vi "Facade 1.vi"(0 "Data In":T8, 2 "Display State In":T2={"Item_Refnums_Array"=[], "Root Command"={"Operation"=enum."Add Item", "Data"=variant}}, 3 "Container State":T7) -> (6 "Data Out":T8, 7 "Display State Out":T2={"Item_Refnums_Array"=[], "Root Command"={"Operation"=enum."Add Item", "Data"=variant}}, 8 "Action":T1)   [LabVIEW 2011, in "Root_XControl.xctl"]
uses:
  Root_XControl.xctl
  Data 1.ctl
  <vilib>/_xctls/Container State.ctl
  State 1.ctl
  Controls/References/Item_Refnums.ctl
  Controls/References/Item_Command_Refnum.ctl
  Controls/Item_Command_Enum.ctl
  Controls/Root_Command.ctl
  Controls/Root_Command_Enum.ctl
  <vilib>/_xctls/Action.ctl
  <vilib>/_xctls/XControlSupport.lvlib
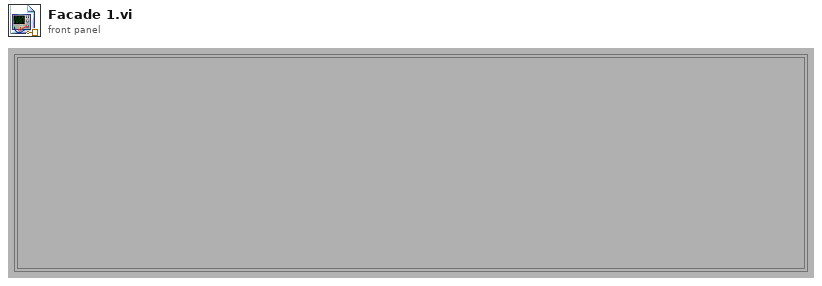
[diagram p1: front panel]
types:
  T1 = typedef "XControlSupport.lvlib/Action.ctl" = cluster{"Data Changed?":bool, "State Changed?":bool, "Action Name":string}
  T2 = typedef "Root_XControl.xctl/State 1.ctl" = cluster{"Item_Refnums_Array":T3[], "Root Command":T5}
  T3 = typedef "Item_Refnums.ctl" = cluster{"VI Refnum":refnum<vi>, "Item_Command_Refnum":T4, "Slide Refnum":refnum<vi>}
  T4 = typedef "Item_Command_Refnum.ctl" = refnum<vi>
  T5 = typedef "Root_Command.ctl" = cluster{"Operation":T6, "Data":variant}
  T6 = typedef "Root_Command_Enum.ctl" = enum16{"Idle", "Add Item", "Delete Item", "Delete All"}
  T7 = typedef "XControlSupport.lvlib/Container State.ctl" = cluster{"Indicator?":bool, "Run Mode?":bool, " Refnum":refnum<vi>}
  T8 = typedef "Root_XControl.xctl/Data 1.ctl" = dbl[]
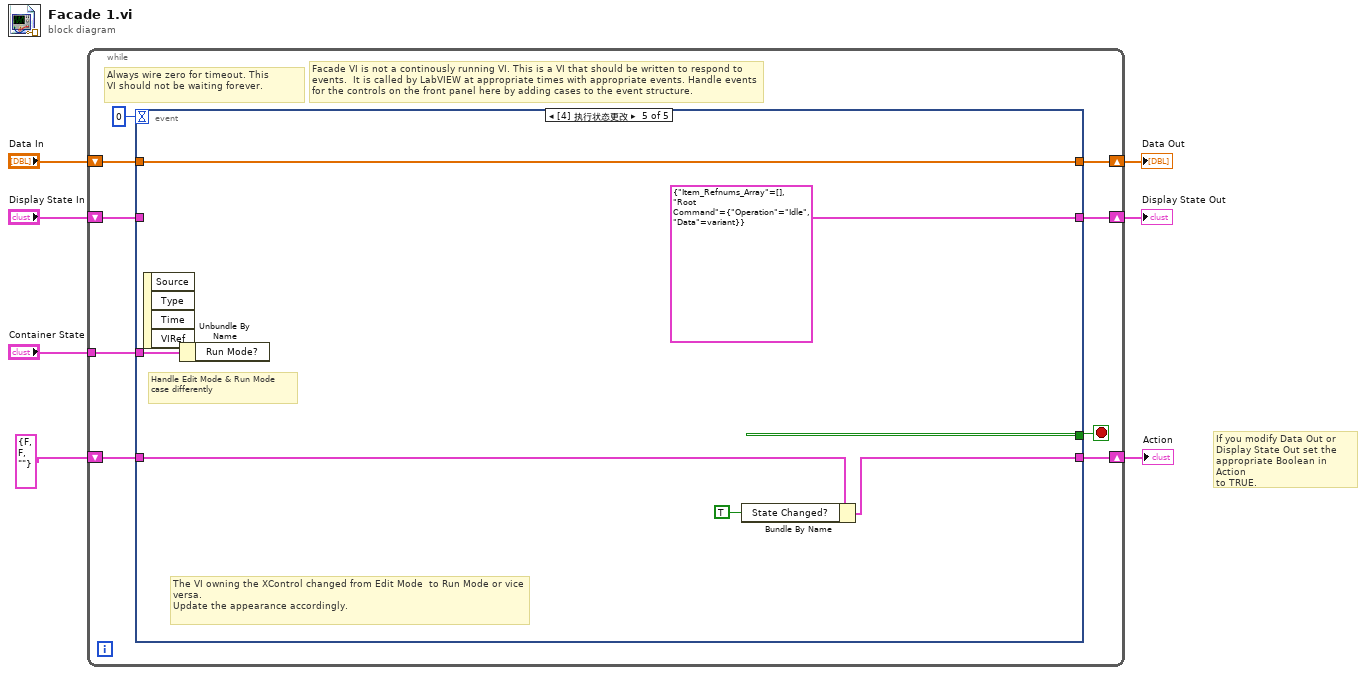
[diagram p0: block diagram]
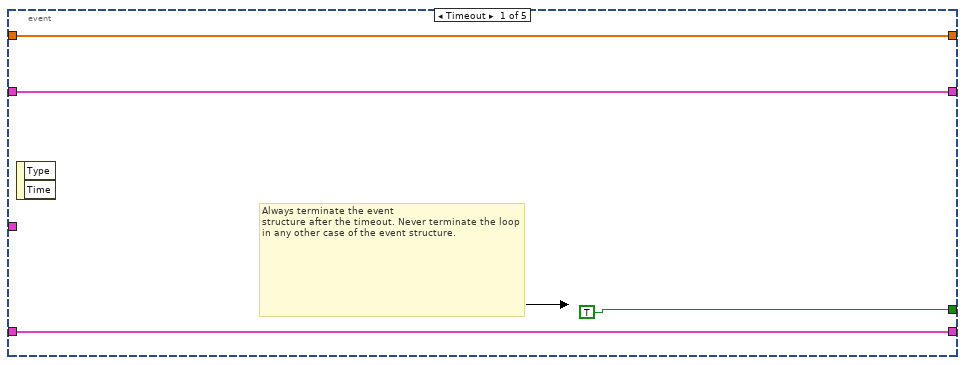
[diagram p2: hidden frame]
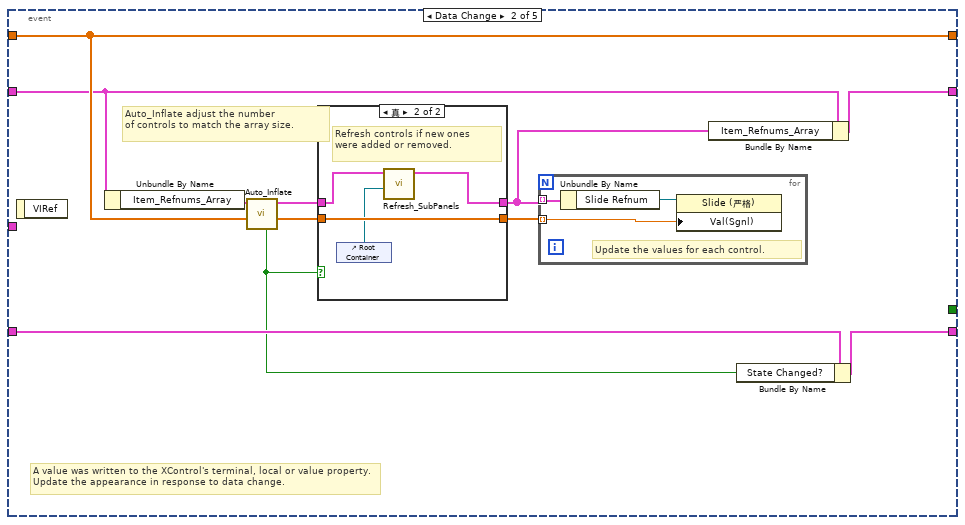
[diagram p3: hidden frame]
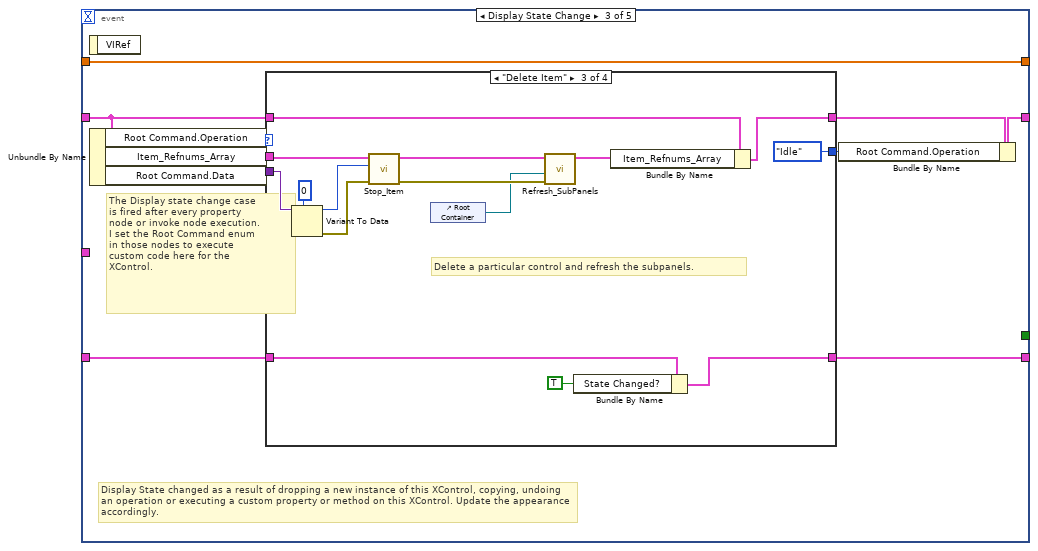
[diagram p5: hidden frame]
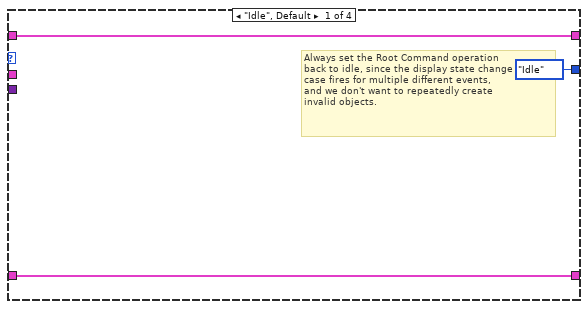
[diagram p6: hidden frame]
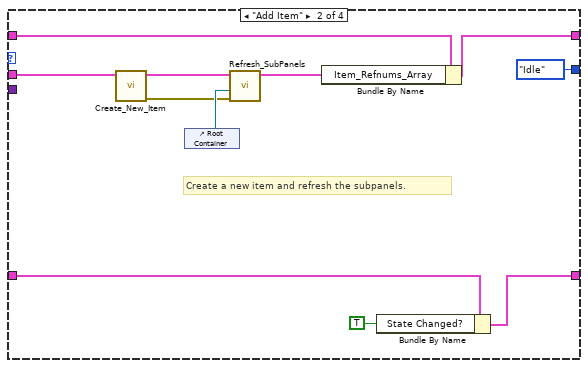
[diagram p7: hidden frame]
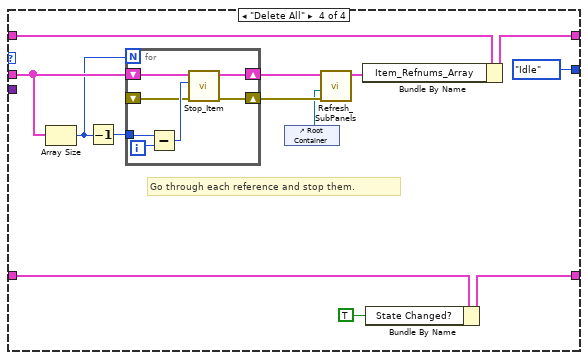
[diagram p8: hidden frame]
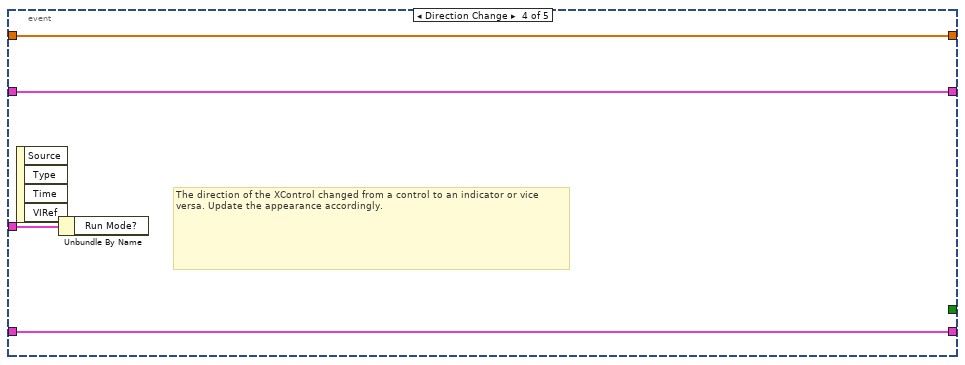
[diagram p9: hidden frame]
diagram:
  # "If you modify Data Out or\nDisplay State Out set the\nappropriate Boolean in Action\nto TRUE."
  n1 = while {
    shift-right: [w15] -> w1
    shift-left: "Display State In" -> [w16]
    tunnel: "Container State" -> [w12]
    shift-right: [w10] -> w7
    shift-left: "Data In" -> [w11]
    shift-right: [w8] -> w3
    shift-left: T1 {"Data Changed?"=FALSE, "State Changed?"=FALSE, "Action Name"=""} ("Action") -> [w9]
    stop <- w14 stop-if-true
    # "Facade VI is not a continously running VI. This is a VI that should be written to respond to events.  It is called by LabVIEW at appropriate times with appropriate events. Handle events for the controls on the front panel here by adding cases to the event structure."
    # "Always wire zero for timeout. This\nVI should not be waiting forever."
    n2 = event shown="[4] 执行状态更改" {
      selector: _ -> [_ _ _ _ _]
      dyn-events: _ -> [_ _ _ _ _]
      timeout: 0 -> [_ _ _ _ _]
      tunnel: w16 -> [w18 w29 w49 w102 _]
      tunnel: [w18 w28 w45 w102 T2 {"Item_Refnums_Array"=[], "Root Command"={"Operation"=enum."Idle", "Data"=variant}} ("Display State In")] -> w15
      tunnel: [TRUE _ _ _ _] -> w14
      tunnel: w12 -> [_ _ _ w103 w109]
      tunnel: w11 -> [w17 w30 w50 w101 w108]
      tunnel: [w17 w30 w50 w101 w108] -> w10
      tunnel: [w19 w26 w46 w100 w105] -> w8
      tunnel: w9 -> [w19 w27 w47 w100 w107]
      event Timeout {
        # "Always terminate the event\nstructure after the timeout. Never terminate the loop in any other case of the event structure."
        n3 = event-data() -> ()  [unwired: 1 in, 2 out]
      }
      event Data Change {
        # "Auto_Inflate adjust the number\nof controls to match the array size."
        # "A value was written to the XControl's terminal, local or value property.\nUpdate the appearance in response to data change."
        n4 = event-data() -> ()  [unwired: 1 in, 1 out]
        n5 = Unbundle By Name(w29) -> ("Item_Refnums_Array"=w31:T3[])
        n6 = call "Auto_Inflate.vi"("Data In"=w30, "Item_Refnums_Array"=w31) -> ("Data Out"=w23:dbl[], "Item_Refnums_Array Out"=w24:T3[], "Inflate/Deflate?"=w25:bool)  [unwired: 7 in]
        n7 = case shown="真" w25 {
          tunnel: w24 -> [w33 w36]
          tunnel: w23 -> [w32 w37]
          tunnel: [w32 w37] -> w22
          tunnel: [w33 w35] -> w21
          frame False {
          }
          frame True {
            # "Refresh controls if new ones\nwere added or removed."
            n8 = control-ref of="Root Container"() -> (w34:refnum<vi>)
            n9 = call "Refresh_SubPanels.vi"("Root Container"=w34, "Item_Refnums_Array"=w36) -> ("Item_Refnums_Array Out"=w35:T3[])  [unwired: 8 in, 1 out]
          }
        }
        n10 = for {
          tunnel: w21 -> [w40] mode=indexing
          tunnel: w22 -> [w38] mode=indexing
          # "Update the values for each control."
          n11 = Unbundle By Name(w40) -> ("Slide Refnum"=w39:refnum<vi>)
          n12 = property class="Slide (严格)"(reference=w39, "Val(Sgnl)"=w38) -> ()  [unwired: 1 in, 2 out]
        }
        n13 = Bundle By Name(cluster=w29, "Item_Refnums_Array"=w21) -> (w28:T2)
        n14 = Bundle By Name(cluster=w27, "State Changed?"=w25) -> (w26:T1)
      }
      event Display State Change {
        # "The Display state change case\nis fired after every property\nnode or invoke node execution.\nI set the Root Command enum\nin those nodes to execute\ncustom code here for the\nXControl."
        # "Display State changed as a result of dropping a new instance of this XControl, copying, undoing an operation or executing a custom property or method on this XControl. Update the appearance accordingly."
        n15 = event-data() -> ()  [unwired: 1 in, 1 out]
        n16 = Unbundle By Name(w49) -> ("Root Command.Operation"=w48:T6, "Item_Refnums_Array"=w43:T3[], "Root Command.Data"=w42:variant)
        n17 = case shown="\"Delete Item\"" w48 {
          tunnel: w49 -> [w53 w64 w78 w84]
          tunnel: w47 -> [w52 w61 w76 w92]
          tunnel: [w53 w63 w77 w82] -> w44
          tunnel: [w52 w60 w74 w90] -> w46
          tunnel: w43 -> [_ w57 w71 w89]
          tunnel: w42 -> [_ _ w73 _]
          tunnel: [Root_Command_Enum."Idle" ("Enum") Root_Command_Enum."Idle" ("Enum") Root_Command_Enum."Idle" ("Enum") Root_Command_Enum."Idle" ("Enum")] -> w41
          frame "Idle", Default {
            # "Always set the Root Command operation\nback to idle, since the display state change\ncase fires for multiple different events,\nand we don't want to repeatedly create\ninvalid objects."
          }
          frame "Add Item" {
            # "Create a new item and refresh the subpanels."
            n18 = call "Create_New_Item.vi"("Item_Refnums_Array In"=w57) -> ("error out"=w54:errorcluster, "Item_Refnums_Array Out"=w56:T3[])  [unwired: 9 in]
            n19 = control-ref of="Root Container"() -> (w58:refnum<vi>)
            n20 = call "Refresh_SubPanels.vi"("error in (no error)"=w54, "Root Container"=w58, "Item_Refnums_Array"=w56) -> ("Item_Refnums_Array Out"=w55:T3[])  [unwired: 7 in, 1 out]
            n21 = Bundle By Name(cluster=w64, "Item_Refnums_Array"=w55) -> (w63:T2)
            n22 = Bundle By Name(cluster=w61, "State Changed?"=TRUE) -> (w60:T1)
          }
          frame "Delete Item" {
            # "Delete a particular control and refresh the subpanels."
            n23 = Variant To Data(type=0, Variant=w73) -> (data=w69:i32, error out=w70:errorcluster)  [unwired: 1 in]
            n24 = call "Stop_Item.vi"("error in (no error)"=w70, "Index"=w69, "Item_Refnums_Array"=w71) -> ("error out"=w67:errorcluster, "Item_Refnums_Array Out"=w68:T3[])  [unwired: 7 in]
            n25 = control-ref of="Root Container"() -> (w65:refnum<vi>)
            n26 = call "Refresh_SubPanels.vi"("error in (no error)"=w67, "Root Container"=w65, "Item_Refnums_Array"=w68) -> ("Item_Refnums_Array Out"=w66:T3[])  [unwired: 7 in, 1 out]
            n27 = Bundle By Name(cluster=w76, "State Changed?"=TRUE ("Data Changed?")) -> (w74:T1)
            n28 = Bundle By Name(cluster=w78, "Item_Refnums_Array"=w66) -> (w77:T2)
          }
          frame "Delete All" {
            # "Go through each reference and stop them."
            n29 = Array Size(array=w89) -> (size(s)=w80:i32)
            n30 = Decrement(x=w80) -> (x-1=w88:i32)
            n31 = for {
              N: w80 -> [_]
              shift-right: [w95] -> w87
              shift-left: w89 -> [w99]
              tunnel: w88 -> [w98]
              shift-right: [w94] -> w86
              shift-left: _ -> [w93]
              i -> [w97]
              n32 = Subtract(x=w98, y=w97) -> (x-y=w96:i32)
              n33 = call "Stop_Item.vi"("error in (no error)"=w93, "Index"=w96, "Item_Refnums_Array"=w99) -> ("error out"=w94:errorcluster, "Item_Refnums_Array Out"=w95:T3[])  [unwired: 7 in]
            }
            n34 = control-ref of="Root Container"() -> (w85:refnum<vi>)
            n35 = call "Refresh_SubPanels.vi"("error in (no error)"=w86, "Root Container"=w85, "Item_Refnums_Array"=w87) -> ("Item_Refnums_Array Out"=w83:T3[])  [unwired: 7 in, 1 out]
            n36 = Bundle By Name(cluster=w84, "Item_Refnums_Array"=w83) -> (w82:T2)
            n37 = Bundle By Name(cluster=w92, "State Changed?"=TRUE) -> (w90:T1)
          }
        }
        n38 = Bundle By Name(cluster=w44, "Root Command.Operation"=w41) -> (w45:T2)
      }
      event Direction Change {
        # "The direction of the XControl changed from a control to an indicator or vice versa. Update the appearance accordingly."
        n39 = event-data() -> ()  [unwired: 1 in, 4 out]
        n40 = Unbundle By Name(w103) -> ()  [unwired: 1 out]
      }
      event Exec State Change {
        # "The VI owning the XControl changed from Edit Mode  to Run Mode or vice versa.\nUpdate the appearance accordingly."
        # "Handle Edit Mode & Run Mode\ncase differently"
        n41 = event-data() -> ()  [unwired: 1 in, 4 out]
        n42 = Unbundle By Name(w109) -> ()  [unwired: 1 out]
        n43 = Bundle By Name(cluster=w107, "State Changed?"=TRUE) -> (w105:T1)
      }
    }
  }
  "Display State Out" <- w1
  "Data Out" <- w7
  "Action" <- w3
